vi "Decode_stream_data.vi"(6 "Error In":errorcluster, 8 "Tare":bool, 9 "Sensor Output - Position (mm) 2":dbl[][](array[numeric]), 11 "Bxyz":dbl[][](array[numeric])) -> (0 "Error Out":errorcluster, 1 "3D Plot lvclass Array out":refnum<class "3D Plot Datatype.lvclass">[](array[class]), 2 "mean 2":dbl, 3 "mean":dbl, 5 "Sensor Output - Position (mm) 3":dbl[][](array[numeric]))   [LabVIEW 2018]
uses:
  <vilib>/Math Plots/3D Math Plots/3D Plot/3D Plot Datatype/3D Plot Datatype.lvclass
  <vilib>/Analysis/baseanly.llb/Mean (DBL).vi
  <vilib>/Math Plots/3D Math Plots/3D Surface/3D Surface Datatype/Public/Plot Helper (Matrix).vi
  <vilib>/Analysis/NI_AALBase.lvlib
  <vilib>/Math Plots/3D Math Plots/3D Surface/3D Surface Datatype/3D Surface Datatype.lvclass
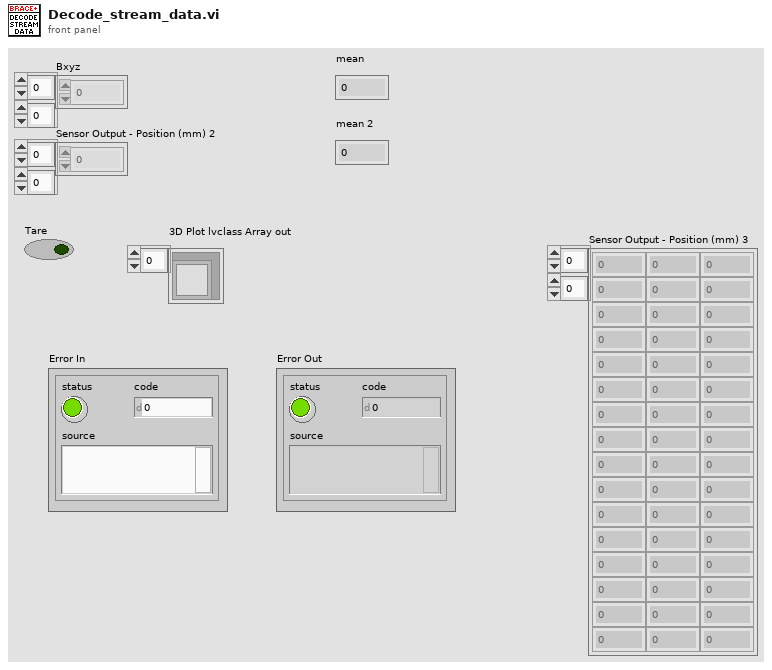
[diagram p1: front panel]
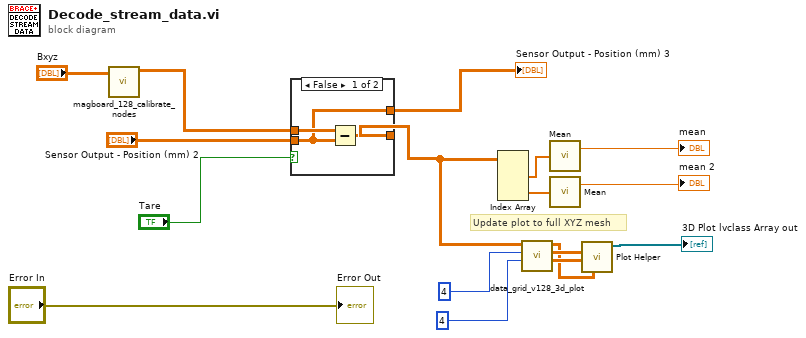
[diagram p0: block diagram]
diagram:
  # "Update plot to full XYZ mesh"
  n1 = call "magboard_128_calibrate_nodes.vi"("Sensor Input (mT)"="Bxyz") -> ("Sensor Output - Position (mm)"=w3:dbl[][])  [unwired: 10 in]
  n2 = case shown="False" "Tare" {
    tunnel: w3 -> [w20 w21]
    tunnel: "Sensor Output - Position (mm) 2" -> [w19 _]
    tunnel: [w19 w21] -> w4
    tunnel: [w18 w21] -> w7
    frame False {
      n3 = Subtract(x=w20, y=w19) -> (x-y=w18:dbl[][])
    }
    frame True {
    }
  }
  "Sensor Output - Position (mm) 3" <- w4
  n4 = Index Array(array=w7) -> (element #1=w16:dbl[], element #2=w17:dbl[])  [unwired: 4 in]
  n5 = call "data_grid_v128_3d_plot.vi"("No. Rows"=4 ("Row Length"), "No. Columns"=4, "Sensor Data"=w7) -> ("Y (GRID)"=w11:dbl[][], "X (GRID)"=w12:dbl[][], "Z (GRID)"=w10:dbl[][])  [unwired: 6 in]
  n6 = call-poly <vilib>:"Mean.vi"("X"=w16) -> ("mean"=→"mean":dbl)  [unwired: 1 out]
  n7 = call-poly <vilib>:"Mean.vi"("X"=w17) -> ("mean"=→"mean 2":dbl)  [unwired: 1 out]
  n8 = call-poly <vilib>:"Plot Helper.vi"("z matrix"=w10, "y matrix"=w11, "x matrix"=w12) -> ("3D Plot lvclass Array out"=→"3D Plot lvclass Array out":refnum<class "3D Plot Datatype.lvclass">[])  [unwired: 3 in, 5 out]
  "Error Out" <- "Error In"
